vi "Load.vi"() -> ()   [LabVIEW 2016]
uses:
  <vilib>/Statechart/Common/IntGuid.ctl
  <vilib>/Statechart/Common/DbgID.ctl
  <vilib>/Statechart/Infrastructure/RTStatechart/RunTime SCN.xnode
  <vilib>/Statechart/Common/NI_SC_LVSCCommonFiles.lvlib
panel:
  in  "用户 4":bool
  in  "用户 3":bool
  in  "用户 2":bool
  in  "用户 1":bool
  out "二维图片":picture
  out "运行状态":string
  in  "停止按钮":bool
  in  "启动按钮":bool
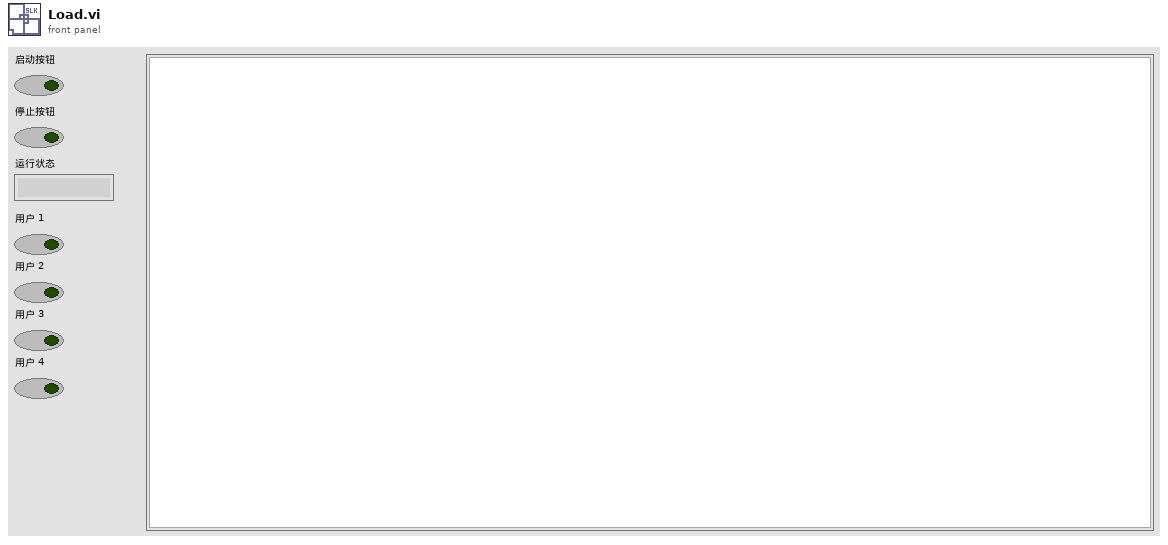
[diagram p1: front panel]
types:
  T1 = typedef "初识状态图-分支的使用-抢答器.lvsc/Inputs.ctl" = cluster{"启动按钮":bool, "停止按钮":bool, "用户 1":bool, "用户 2":bool, "用户 3":bool, "用户 4":bool}
  T2 = typedef "NI_SC_LVSCCommonFiles.lvlib/IntGuid.ctl" = cluster{"Data1":u32, "Data2":u16, "Data3":u16, "Data4":u8, "Data5":u8, "Data6":u8, "Data11":u8, "Data9":u8, "Data10":u8, "Data8":u8, "Data7":u8}
  T3 = typedef "NI_SC_LVSCCommonFiles.lvlib/DbgID.ctl" = cluster{"VIRef":u32, "IntGUID":T2}
  T4 = typedef "初识状态图-分支的使用-抢答器.lvsc/Outputs.ctl" = cluster{"执行状态":string}
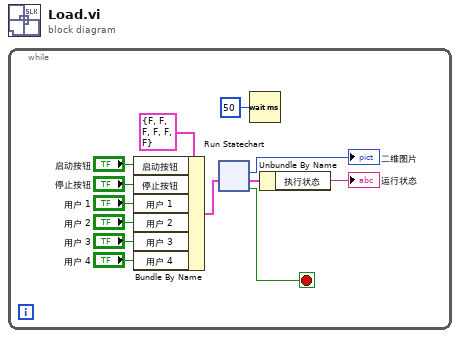
[diagram p0: block diagram]
diagram:
  n1 = while {
    stop <- w6 stop-if-true
    n2 = Bundle By Name(cluster=T1 {"启动按钮"=FALSE, "停止按钮"=FALSE, "用户 1"=FALSE, "用户 2"=FALSE, "用户 3"=FALSE, "用户 4"=FALSE} ("Inputs"), "启动按钮"="启动按钮", "停止按钮"="停止按钮", "用户 1"="用户 1", "用户 2"="用户 2", "用户 3"="用户 3", "用户 4"="用户 4") -> (w10:T1)
    n3 = xnode "Run Statechart"("Inputs"=w10) -> ("Terminated?"=w6:bool, "Outputs"=w9:T4, "Diagram Display"=→"二维图片":picture)  [unwired: 3 in]
    n4 = Wait (ms)(milliseconds to wait=u32 50 ("等待时间（毫秒）")) -> ()  [unwired: 1 out]
    n5 = Unbundle By Name(w9) -> ("执行状态"=→"运行状态":string)
  }
